vi "templates analysis HEADER data keys.vi"(9 "Template Keys":T1, 10 "HTM Keys":T1) -> (2 "HTM Keys":T1)   [LabVIEW 2011]
uses:
  Addons/internet/utils/keyedarr.llb/Keyed Array.ctl
  Addons/internet/utils/strutil.llb/Case Matching.ctl
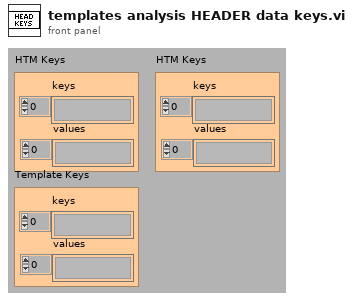
[diagram p1: front panel]
types:
  T1 = typedef "Keyed Array.ctl" = cluster{"keys":string[], "values":string[]}
  T2 = typedef "Case Matching.ctl" = enum16{"a != A", "a == A", "system"}
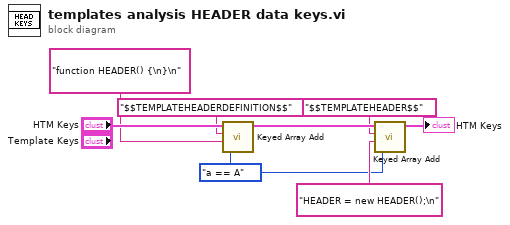
[diagram p0: block diagram]
diagram:
  w1 = Case_Matching."a == A" ("case matching (sensitive)")
  n1 = call "Keyed Array Add.vi"("case matching (sensitive)"=w1, "value"="function HEADER() {\n}\n", "key"="$$TEMPLATEHEADERDEFINITION$$", "array in"="HTM Keys") -> ("array out"=w5:T1)  [unwired: 3 out]
  n2 = call "Keyed Array Add.vi"("case matching (sensitive)"=w1, "value"="HEADER = new HEADER();\n", "key"="$$TEMPLATEHEADER$$", "array in"=w5) -> ("array out"=→"HTM Keys":T1)  [unwired: 3 out]
